vi "Cleanup.vi"(8 "error in (no error)":errorcluster, 9 "JSON":string, 10 "Owner":refnum<vi>, 11 "vi refnum":refnum<vi>) -> (0 "error out":errorcluster, 2 "JSON out":string, 3 "Type out":variant)   [LabVIEW 2018, in "JSON to LVConstant Test.lvlib"]
uses:
  JSON to LVConstant Test.lvlib
  897828fa-4a40-4be3-9934-cd31794559d2.vi
  ab42581f-ee8f-4c1a-bdc7-247f6cbec308.vi
  <vilib>/JDP Science/JSONtext/JSON text to Variant.vi
  <vilib>/JDP Science/JSONtext/Variant to JSON Text.vi
  <vilib>/JDP Science/JSONtext/LVClass Serializer/JSONtext LVClass Serializer.lvclass
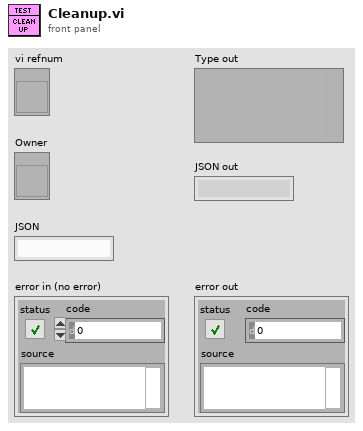
[diagram p1: front panel]
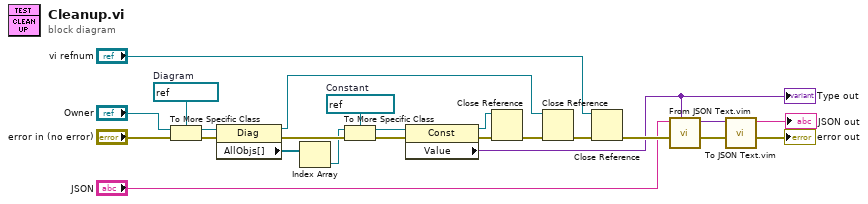
[diagram p0: block diagram]
diagram:
  w21 = refnum<vi> refnum  # Constant
  w15 = refnum<vi> refnum  # Diagram
  n1 = To More Specific Class(target class=w15, reference="Owner", error in="error in (no error)") -> (specific class reference=w14:refnum<vi>, error out=w12:errorcluster)
  n2 = property on="Property Node" class="Diag"(reference=w14, error in=w12) -> (reference out=w11:refnum<vi>, error out=w24:errorcluster, "AllObjs[]"=w16:refnum<vi>[])
  n3 = Index Array(array=w16) -> (element=w19:refnum<vi>)  [unwired: 1 in]
  n4 = To More Specific Class(target class=w21, reference=w19, error in=w24) -> (specific class reference=w20:refnum<vi>, error out=w18:errorcluster)
  n5 = property on="Property Node" class="Const"(reference=w20, error in=w18) -> (reference out=w22:refnum<vi>, error out=w17:errorcluster, "Value"=w2:variant)
  "Type out" <- w2
  n6 = Close Reference(reference=w22, error in (no error)=w17) -> (error out=w23:errorcluster)
  n7 = Close Reference(reference=w11, error in (no error)=w23) -> (error out=w9:errorcluster)
  n8 = Close Reference(reference="vi refnum", error in (no error)=w9) -> (error out=w7:errorcluster)
  n9 = call "From JSON Text.vim"("Data Type and Default Value"=w2, "error in (no error)"=w7, "JSON"="JSON") -> ("error out"=w6:errorcluster, "Data out"=w3:variant)  [unwired: 7 in]
  n10 = call "To JSON Text.vim"("error in (no error)"=w6, "Anything"=w3) -> ("error out"=→"error out":errorcluster, "<JSON>"=→"JSON out":string)  [unwired: 8 in]
